vi "Equip-Get config list.vi"(11 "error in (no error)":errorcluster) -> (4 "section names":string[](array[string]), 6 "active index":i32, 14 "active config":string, 15 "error out":errorcluster)   [LabVIEW 2015]
uses:
  <vilib>/Utility/config.llb/Read Key (String).vi
  <vilib>/Utility/config.llb/NI_LVConfig.lvlib
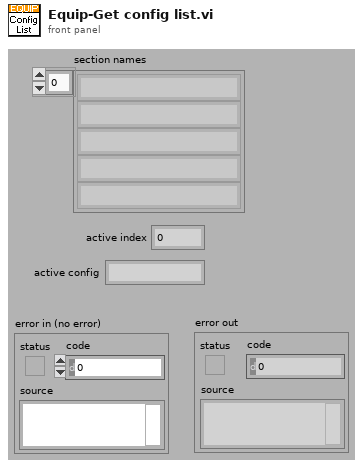
[diagram p1: front panel]
types:
  T1 = typedef "NI_LVConfig.lvlib/Config Data RefNum.ctl" = refnum<k1>
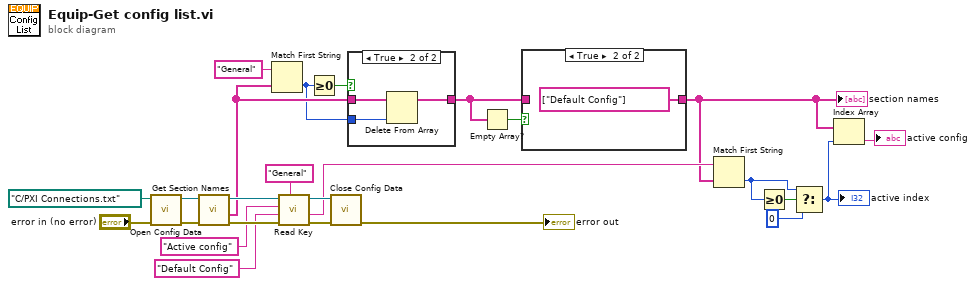
[diagram p0: block diagram]
diagram:
  n1 = call <vilib>:"Open Config Data.vi"("error in (no error)"="error in (no error)", "configuration file path"=path "C:/PXI Connections.txt") -> ("error out"=w23:errorcluster, "refnum"=w22:T1)  [unwired: 7 in, 1 out]
  n2 = call <vilib>:"Get Section Names.vi"("error in (no error)"=w23, "refnum"=w22) -> ("error out"=w21:errorcluster, "section names"=w12:string[], "refnum out"=w16:T1)  [unwired: 7 in]
  n3 = Match First String(2:w12, 3:"General" ("string")) -> (0:w11:i32)  [unwired: 1 out]
  n4 = call-poly <vilib>:"Read Key.vi"("section"="General", "error in (no error)"=w21, "default value"="Default Config" ("key"), "key"="Active config", "refnum"=w16) -> ("error out"=w20:errorcluster, "value"=w7:string, "refnum out"=w15:T1)  [unwired: 3 in, 1 out]
  n5 = Greater Or Equal To 0?(x=w11) -> (x >= 0?=w13:bool)
  n6 = call <vilib>:"Close Config Data.vi"("error in (no error)"=w20, "refnum"=w15) -> ("error out"=→"error out":errorcluster)  [unwired: 8 in, 1 out]
  n7 = case shown="True" w13 {
    tunnel: w12 -> [w26 w29]
    tunnel: w11 -> [_ w28]
    tunnel: [w26 w27] -> w8
    frame False {
    }
    frame True {
      n8 = Delete From Array(array=w29, index=w28) -> (array with subset deleted=w27:string[])  [unwired: 1 in, 1 out]
    }
  }
  n9 = Empty Array?(array=w8) -> (empty?=w9:bool)
  n10 = case shown="True" w9 {
    tunnel: [w30 string[] ["Default Config"] ("section names")] -> w3
    tunnel: w8 -> [w30 _]
    frame False {
    }
    frame True {
    }
  }
  "section names" <- w3
  n11 = Match First String(2:w3, 3:w7) -> (0:w5:i32)  [unwired: 1 out]
  n12 = Greater Or Equal To 0?(x=w5) -> (x >= 0?=w6:bool)
  n13 = Select(t=w5, s=w6, f=0) -> (s? t:f=w2:i32)
  "active index" <- w2
  n14 = Index Array(array=w3, index=w2) -> (element=→"active config":string)
